vi "StopLoggingChannels.vi"(8 "error in (no error)":errorcluster, 10 "Data Log Configuration Name":string="Log", 11 "VeriStand Test Case in":refnum<class "VeriStandTestCase.lvclass">) -> (0 "error out":errorcluster, 3 "VeriStand Test Case out":refnum<class "VeriStandTestCase.lvclass">)   [LabVIEW 2015, in "VeriStandTestCase.lvclass"]
uses:
  VeriStandTestCase.lvclass
  VeriStandTestCase.lvclass/VeriStandTestCase.ctl
  <vilib>/NI VeriStand/Execution/Workspace/NI_VS Workspace ExecutionAPI.lvlib
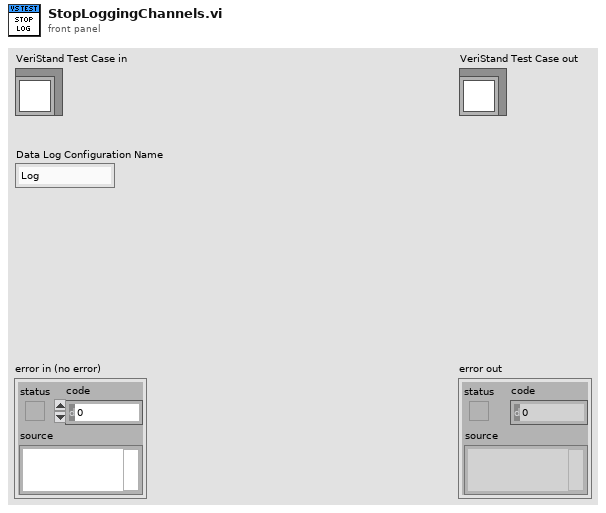
[diagram p1: front panel]
types:
  T1 = typedef "NI_VS Workspace ExecutionAPI.lvlib/WorkspaceAPI.ctl" = refnum<k24>
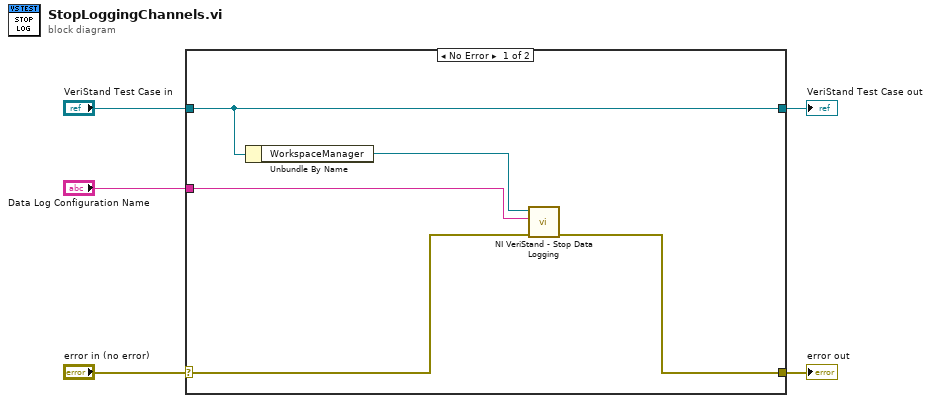
[diagram p0: block diagram]
diagram:
  n1 = case shown="No Error" "error in (no error)" {
    selector: "error in (no error)" -> [w10 w12]
    tunnel: [w9 w12] -> w4
    tunnel: [w8 w11] -> w2
    tunnel: "VeriStand Test Case in" -> [w8 w11]
    tunnel: "Data Log Configuration Name" -> [w6 _]
    frame No Error {
      n2 = Unbundle By Name(w8) -> ("WorkspaceManager"=w7:T1)
      n3 = call <vilib>:"NI VeriStand - Stop Data Logging.vi"("error in (no error)"=w10, "Data Log Configuration Name"=w6, "WorkspaceManager in"=w7) -> ("error out"=w9:errorcluster)  [unwired: 7 in, 1 out]
    }
    frame Error {
    }
  }
  "error out" <- w4
  "VeriStand Test Case out" <- w2
